vi "PH_HamamatsuCamera.set ROI.vi"(0 "VI in":refnum<vi>, 2 "IMAQ1394 Session In in":T3, 3 "Attribute Information Array":T2(array[cluster]), 5 "error in (no error)":errorcluster) -> (14 "VI out":refnum<vi>, 16 "IMAQ1394 Session In out":T3, 19 "error out":errorcluster)   [LabVIEW 2014]
doc: "This VI reads the Cam attributes \"Left\", \"Right\", \"Bottom\" and \"Top\" from the cam and sets them to class attributes as well as to the related GUI elements."
uses:
  PH_HamamatsuCamera.lvlib
  <vilib>/userdefined/High Color/IMAQdx.ctl
  <vilib>/vision/driver/IMAQdx.llb/IMAQdx Attribute Type.ctl
  <vilib>/vision/driver/NI_Vision_Acquisition_Software.lvlib
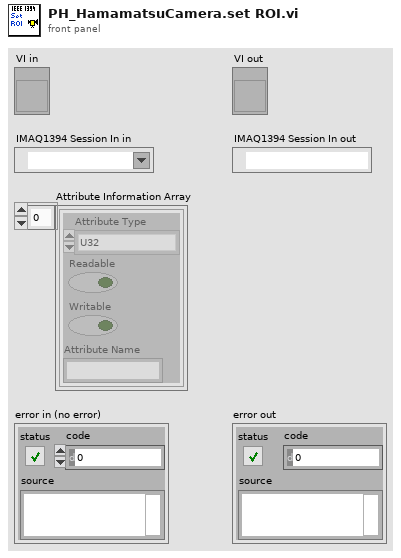
[diagram p1: front panel]
types:
  T1 = typedef "NI_Vision_Acquisition_Software.lvlib/IMAQdx Attribute Type.ctl" = enum32{"U32", "I64", "DBL", "String", "Enum", "Bool", "Command"}
  T2 = cluster{"Attribute Type":T1, "Readable":bool, "Writable":bool, "Attribute Name":string}[]
  T3 = typedef "IMAQdx.ctl" = refnum<k21>
  T4 = typedef "PH_HamamatsuCamera.lvlib/PH_HamamatsuCamera.i attribute.ctl" = cluster{"Gui Refs":cluster{"Frame Rate":refnum<vi>, "Get Frame Rate":refnum<vi>, "Camera State":refnum<vi>, "Start Cam":refnum<vi>, "Show Image":refnum<vi>, "Get Histogram":refnum<vi>, "Mapping":refnum<vi>, "Histogram":refnum<vi>, "Center Cross":refnum<vi>, "Center of Gravity":refnum<vi>, "Scale Factor [%]":refnum<vi>, "Save Image":refnum<vi>, "Palette":refnum<vi>, "Connect":refnum<vi>, "Camera State Bar":refnum<vi>, "Cam Error":refnum<vi>, "Camera Details":refnum<vi>, "ROI":refnum<vi>, "Set ROI to Maximum":refnum<vi>, "Trigger Parameters":refnum<vi>, "Brightness":refnum<vi>, "Shutter":refnum<vi>, "Gain":refnum<vi>, "Trigger Timeout":refnum<vi>, "Subtract Background":refnum<vi>, "Cam List":refnum<vi>, "Parameters":refnum<vi>, "Trigger Polarity":refnum<vi>, "Trigger Mode":refnum<vi>}, "Cam":cluster{"State":T5, "Restart":bool, "Source Notifier":refnum<notifier>, "Handle":i32, "Details":cluster{"Model":string, "Camera ID":string, "Firmware":string}, "Error":errorcluster, "Buffer Info":cluster{"height":u32, "width":u32, "datatype":u32}}, "Images":cluster{"CamI16":T6, "OperationI16":T6, "PSDB I16":T6}, "Window Image":cluster{"Indicate Image":bool, "Window No.":i32, "Scale Facor":dbl, "Center Cross":bool, "Subtract Backgr":bool, "CoG":bool, "Color Palette":cluster{"Red":u8, "Green":u8, "Blue":u8}[], "Image On":bool}, "Default Prdc Int":i32, "Performance":cluster{"on":bool, "Timestamp Last Frame":i32}, "Histogram":cluster{"on":bool, "Mapping":bool}, "Save Image":cluster{"Save":bool, "File refnum":refnum<file>}, "Setting Service ID":i32, "GUI Manager Path":string, "Screen":cluster{"x-resolution":i16, "y-resolution":i16}, "Image Position Path":string, "H Offset":cluster{"Value":i32, "Minimum":i32, "Maximum":i32, "Increment":i32}, "V Offset":cluster{"Value":i32, "Minimum":i32, "Maximum":i32, "Increment":i32}, "H Width":cluster{"Value":i32, "Minimum":i32, "Maximum":i32, "Increment":i32}, "V Width":cluster{"Value":i32, "Minimum":i32, "Maximum":i32, "Increment":i32}, "Trigger Parameters":cluster{"Mode":u32, "Polarity":u32, "Times":u32, "Delay":dbl}, "Trigger Timeout":u32, "Parameters":T7[], "Cam Setting Parameters":cluster{"Brightness":string, "Shutter":string, "Gain":string}}
  T5 = typedef "Device State.ctl" = i32
  T6 = typedef "IMAQ Image.ctl" = refnum<image>
  T7 = typedef "PH_HamamatsuCamera.lvlib/PH_HamamatsuCamera.Parameter Set.ctl" = cluster{"Name":string, "Value":dbl, "Range":cluster{"min":dbl, "max":dbl, "step":dbl}}
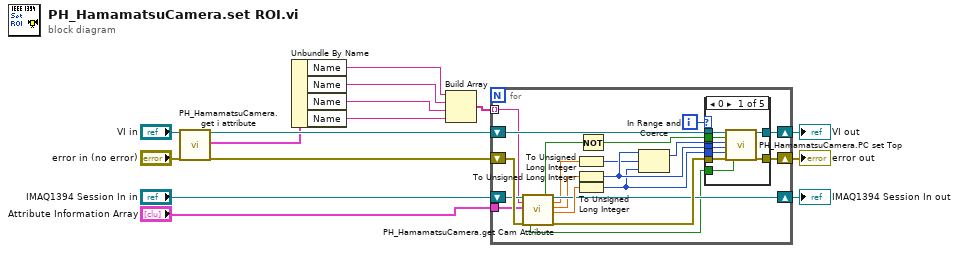
[diagram p0: block diagram]
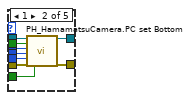
[diagram p2: hidden frame]
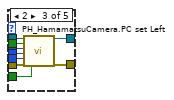
[diagram p3: hidden frame]
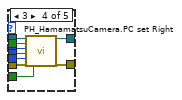
[diagram p4: hidden frame]
diagram:
  n1 = call "PH_HamamatsuCamera.get i attribute.vi"("i ref in"="VI in", "error in (no error)"="error in (no error)") -> ("i ref out"=w4:refnum<vi>, "i attribute"=w2:T4, "error out"=w3:errorcluster)  [unwired: 15 in]
  n2 = Unbundle By Name(w2) -> ("Name"=w5:string, "Name"=w6:string, "Name"=w7:string, "Name"=w8:string)
  n3 = Build Array(w5, w6, w7, w8) -> (w1:string[])
  n4 = for {
    tunnel: w1 -> [w28] mode=indexing
    shift-right: [w23] -> w15
    shift-left: "IMAQ1394 Session In in" -> [w29]
    shift-right: [w35] -> w12
    shift-left: w3 -> [w30]
    shift-right: [w33] -> w10
    shift-left: w4 -> [w34]
    tunnel: "Attribute Information Array" -> [w24]
    i -> [w32]
    n5 = call "PH_HamamatsuCamera.get Cam Attribute.vi"("IMAQ1394 Session In"=w29, "Cam Number Attribute Name"=w28, "Attribute Information Array"=w24, "error in (no error)"=w30) -> ("Attribute writable?"=w21:bool, "Attribute read?"=w27:bool, "IMAQ1394 Session Out"=w23:T3, "Current Num Value"=w20:dbl, "Maximum"=w22:dbl, "Minimum"=w25:dbl, "error out"=w31:errorcluster)  [unwired: 2 in, 7 out]
    n6 = To Unsigned Long Integer(number=w20) -> (unsigned 32bit integer=w17:u32)
    n7 = To Unsigned Long Integer(number=w22) -> (unsigned 32bit integer=w19:u32)
    n8 = To Unsigned Long Integer(number=w25) -> (unsigned 32bit integer=w18:u32)
    n9 = Not(x=w27) -> (.not. x?=w26:bool)
    n10 = In Range and Coerce(upper limit=w19, x=w17, lower limit=w18) -> (coerced(x)=w16:u32)  [unwired: 1 out]
    n11 = case shown="0" w32 {
      tunnel: w31 -> [w42 w53 w62 w71 w73]
      tunnel: [w41 w52 w61 w70 w73] -> w35
      tunnel: w34 -> [w44 w51 w60 w69 w72]
      tunnel: [w43 w50 w59 w68 w72] -> w33
      tunnel: w16 -> [w36 w45 w54 w63 _]
      tunnel: w26 -> [w40 w49 w58 w67 _]
      tunnel: w19 -> [w38 w48 w57 w66 _]
      tunnel: w18 -> [w37 w47 w56 w65 _]
      tunnel: w21 -> [w39 w46 w55 w64 _]
      frame 0 {
        n12 = call "PH_HamamatsuCamera.PC set Top.vi"("i ref in"=w44, "No Info? (False)"=w40, "Top"=w36, "Maximum Top"=w38, "Minimum Top"=w37, "error in (no error)"=w42, "Top writable? (True)"=w39) -> ("i ref out"=w43:refnum<vi>, "error out"=w41:errorcluster)  [unwired: 10 in, 1 out]
      }
      frame 1 {
        n13 = call "PH_HamamatsuCamera.PC set Bottom.vi"("i ref in"=w51, "No Info? (False)"=w49, "Bottom"=w45, "Maximum Bottom"=w48, "Minimum Bottom"=w47, "error in (no error)"=w53, "Bottom writable? (True)"=w46) -> ("i ref out"=w50:refnum<vi>, "error out"=w52:errorcluster)  [unwired: 10 in, 1 out]
      }
      frame 2 {
        n14 = call "PH_HamamatsuCamera.PC set Left.vi"("i ref in"=w60, "No Info? (False)"=w58, "Left"=w54, "Maximum Left"=w57, "Minimum Left"=w56, "error in (no error)"=w62, "Left writable? (True)"=w55) -> ("i ref out"=w59:refnum<vi>, "error out"=w61:errorcluster)  [unwired: 10 in, 1 out]
      }
      frame 3 {
        n15 = call "PH_HamamatsuCamera.PC set Right.vi"("i ref in"=w69, "No Info? (False)"=w67, "Right"=w63, "Maximum Right"=w66, "Minimum Right"=w65, "error in (no error)"=w71, "Right writable? (True)"=w64) -> ("i ref out"=w68:refnum<vi>, "error out"=w70:errorcluster)  [unwired: 10 in, 1 out]
      }
      frame Default {
      }
    }
  }
  "IMAQ1394 Session In out" <- w15
  "error out" <- w12
  "VI out" <- w10
